vi "InitializeAccessorVIs.vi"(8 "error in (no error)":errorcluster, 11 "ClassReflector in":refnum<class "ClassReflector.lvclass">) -> (0 "error out":errorcluster, 3 "ClassReflector out":refnum<class "ClassReflector.lvclass">)   [LabVIEW 2023, in "ClassReflector.lvclass"]
uses:
  ClassReflector.lvclass
  ClassReflector.lvclass/ClassReflector.ctl
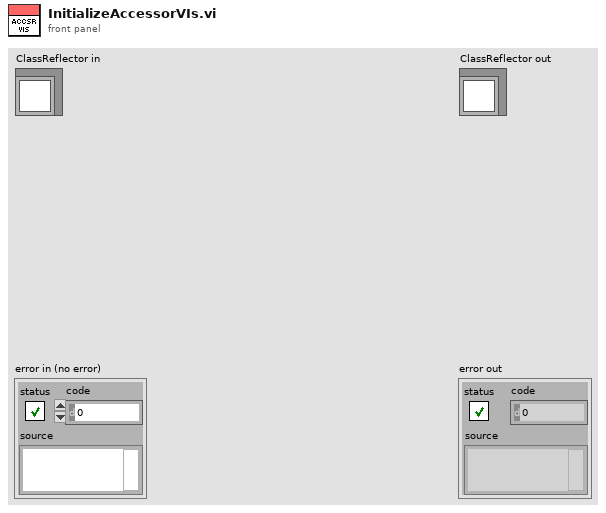
[diagram p1: front panel]
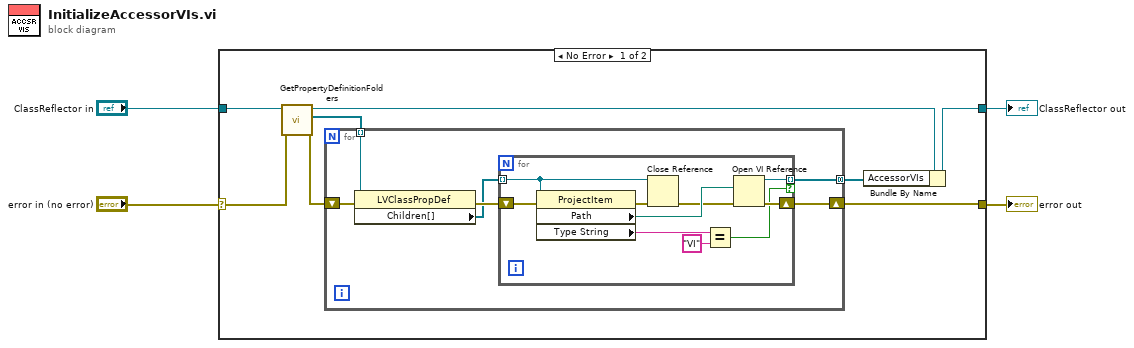
[diagram p0: block diagram]
diagram:
  n1 = case shown="No Error" "error in (no error)" {
    selector: "error in (no error)" -> [w11 w30]
    tunnel: [w8 w30] -> w3
    tunnel: [w6 w29] -> w1
    tunnel: "ClassReflector in" -> [w12 w29]
    frame No Error {
      n2 = call "GetPropertyDefinitionFolders.vi"("error in (no error)"=w11, "ClassReflector in"=w12) -> ("error out"=w9:errorcluster, "PropertyDefinitionFolders"=w10:refnum<vi>[], "ClassReflector out"=w7:refnum<class "ClassReflector.lvclass">)  [unwired: 7 in]
      n3 = for {
        tunnel: w10 -> [w14] mode=indexing
        shift-right: [w16] -> w8
        shift-left: w9 -> [w18]
        tunnel: [w15] -> w5 mode=concatenating
        n4 = property class="LVClassPropDef"(reference=w14, error in=w18) -> (error out=w17:errorcluster, "Children[]"=w13:refnum<vi>[])  [unwired: 1 out]
        n5 = for {
          shift-right: [w25] -> w16
          shift-left: w17 -> [w26]
          tunnel: [w23] -> w15 mode=indexing if=w22
          tunnel: w13 -> [w19] mode=indexing
          n6 = property class="ProjectItem"(reference=w19, error in=w26) -> (error out=w21:errorcluster, "Path"=w24:path, "Type String"=w28:string)  [unwired: 1 out]
          n7 = Close Reference(reference=w19, error in (no error)=w21) -> (error out=w20:errorcluster)
          n8 = Equal?(x=w28, y="VI") -> (x = y?=w22:bool)
          n9 = Open VI Reference(vi path=w24, error in (no error)=w20) -> (vi reference=w23:refnum<vi>, error out=w25:errorcluster)  [unwired: 4 in]
        }
      }
      n10 = Bundle By Name(cluster=w7, "AccessorVIs"=w5) -> (w6:refnum<class "ClassReflector.lvclass">)
    }
    frame Error {
    }
  }
  "error out" <- w3
  "ClassReflector out" <- w1
